vi "Reset.vi"(8 "error in (no error)":errorcluster, 11 "Impot in":refnum<class "Impot.lvclass">) -> (0 "error out":errorcluster, 3 "Impot out":refnum<class "Impot.lvclass">)   [LabVIEW 2023, in "Impot.lvclass"]
uses:
  Impot.lvclass
  ID/ID.lvclass
  Impot.lvclass/Impot.ctl
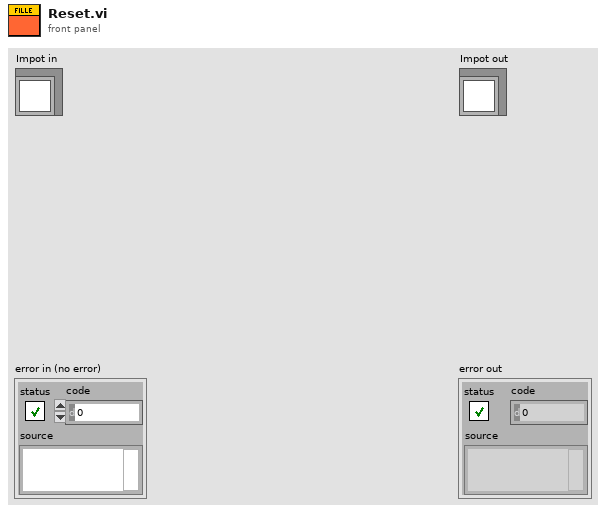
[diagram p1: front panel]
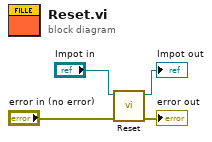
[diagram p0: block diagram]
diagram:
  n1 = call-parent "Reset.vi"("error in (no error)"="error in (no error)", "ID in"="Impot in") -> ("error out"=→"error out":errorcluster, "ID out"=→"Impot out":refnum<class "Impot.lvclass">)  [unwired: 8 in]
